vi "Build Data Folder File Path.vi"() -> (3 "Data Folder File Path":path)   [LabVIEW 2019, in "SEECD System Explorer.lvlib"]
uses:
  SEECD System Explorer.lvlib
  <vilib>/Utility/sysdir.llb/System Directory Type.ctl
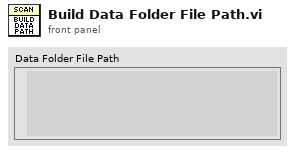
[diagram p1: front panel]
types:
  T1 = typedef "System Directory Type.ctl" = i32
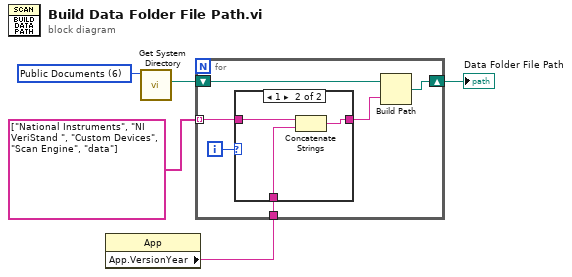
[diagram p0: block diagram]
diagram:
  w5 = T1 6 items=["User Home"=0, "User Desktop"=1, "User Documents"=2, "User Application Data"=3, "User Preferences"=4, "User Temporary"=5, "Public Documents"=6, "Public Application Data"=7, "Public Preferences"=8, "Public Cache"=13, "System Core Libraries"=9, "System Installed Libraries"=10, "Application Files"=11, "Boot Volume Root"=12] ("system directory type")
  n1 = property class="App"() -> ("App.VersionYear"=w2:string)  [unwired: 2 in, 2 out]
  n2 = call <vilib>:"Get System Directory.vi"("system directory type"=w5) -> ("system directory"=w4:path)  [unwired: 10 in]
  n3 = for {
    shift-right: [w10] -> w1
    shift-left: w4 -> [w11]
    tunnel: string[] ["National Instruments", "NI VeriStand ", "Custom Devices", "Scan Engine", "data"] -> [w7] mode=indexing
    tunnel: w2 -> [w6]
    i -> [w9]
    n4 = case shown="1" w9 {
      tunnel: [w12 w14] -> w8
      tunnel: w7 -> [w12 w15]
      tunnel: w6 -> [_ w13]
      frame Default {
      }
      frame 1 {
        n5 = Concatenate Strings(w15, w13) -> (w14:string)
      }
    }
    n6 = Build Path(base path=w11, name or relative path=w8) -> (appended path=w10:path)
  }
  "Data Folder File Path" <- w1
